vi "compress.vi"   [LabVIEW 2015, in "lv-bin-7zip.lvlib" / "v1.lvlib"]
doc: "this vi can be used to create an archive providing the \"source\" folder to populate the archive as well as the archive name. It's as intelligent as the 7zip application, depending on the archive extension you give, it will create an archive with the appropriate extension (i.e. zip, 7z, tar, gz). If no archive is provided, it will prompt you to select a new or existing file. If a folder is given, it will add the contents of the folder."
uses:
  v1.lvlib
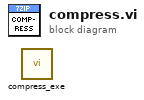
[diagram p0: block diagram]
diagram:
  n1 = call "compress_exe.vi"() -> ()  [unwired: 10 in, 2 out]
